vi "Begin.vi"(8 "error in":errorcluster) -> (0 "error out":errorcluster)   [LabVIEW 2014]
doc: "Called before other user functions, this VI is expected to open initial I/O refnums, load in file data, and do all program initialization. Notice that the <B>error out</B> terminal is simply used for data flow. Wiring it to other structures or subVIs ensures that this VI runs first."
uses:
  <vilib>/Rock Robotics/WPI/SafetyOutput/WPI_SafetyOutputConfigMenu.ctl
  <vilib>/Rock Robotics/WPI/DriverStation/WPI_DriverStationRobotMode2.ctl
  <vilib>/Rock Robotics/WPI/Joystick/WPI_JoystickDeviceEnum.ctl
  <vilib>/Rock Robotics/SystemInterfaces/DIO/FPGA_DIOPWMChannel.ctl
  <vilib>/Rock Robotics/WPI/Solenoid/WPI_SolenoidChannel.ctl
  navX-MXP Library/COMMON/TypeDefs/Value TypeDefs/navX Update Rate.ctl
  navX-MXP Library/COMMON/TypeDefs/Value TypeDefs/navX Interface Protocol.ctl
  <vilib>/Rock Robotics/SystemInterfaces/i2clib/i2c_bus.ctl
  <vilib>/Rock Robotics/SystemInterfaces/DIO/FPGA_DIOChannel.ctl
  <vilib>/Rock Robotics/WPI/Solenoid/WPI_SolenoidValue.ctl
  Robot Global Data.vi
  <vilib>/Rock Robotics/Network Tables/SD Write String Array.vi
  <vilib>/Rock Robotics/WPI/RobotDrive/WPI_RobotDriveOpen4MotorWithTalon.vi
  <vilib>/Rock Robotics/WPI/Solenoid/WPI_SolenoidOpenDouble.vi
  <vilib>/Rock Robotics/WPI/MotorControl/WPI_MotorControlOpen Talon.vi
  <vilib>/Rock Robotics/WPI/Solenoid/WPI_SolenoidSetEnum.vi
  navX-MXP Library/navX-MXP IMU.lvlib
panel:
  out "North":dbl
  out "Opened?":bool
  # "EDITED: 3/8/15"
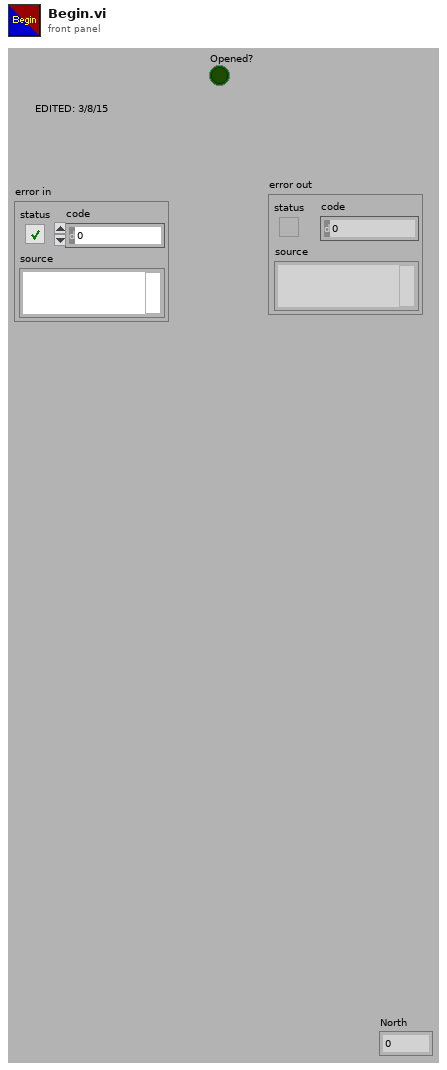
[diagram p1: front panel]
types:
  T1 = typedef "WPI_SolenoidValue.ctl" = enum16{"Off", "On", "Forward", "Reverse"}
  T2 = typedef "WPI_SolenoidChannel.ctl" = enum8{"Solenoid 0", "Solenoid 1", "Solenoid 2", "Solenoid 3", "Solenoid 4", "Solenoid 5", "Solenoid 6", "Solenoid 7", "Invalid"}
  T3 = typedef "FPGA_DIOPWMChannel.ctl" = enum8{"PWM 0", "PWM 1", "PWM 2", "PWM 3", "PWM 4", "PWM 5", "PWM 6", "PWM 7", "PWM 8", "PWM 9", "PWM MXP 0", "PWM MXP 1", "PWM MXP 2", "PWM MXP 3", "PWM MXP 4", "PWM MXP 5", "PWM MXP 6", "PWM MXP 7", "PWM MXP 8", "PWM MXP 9", "Invalid"}
  T4 = typedef "WPI_JoystickDeviceEnum.ctl" = enum16{"USB 0", "USB 1", "USB 2", "USB 3", "USB 4", "USB 5"}
  T5 = typedef "FPGA_DIOChannel.ctl" = enum8{"DIO 0", "DIO 1", "DIO 2", "DIO 3", "DIO 4", "DIO 5", "DIO 6", "DIO 7", "DIO 8", "DIO 9", "DIO MXP 0", "DIO MXP 1", "DIO MXP 2", "DIO MXP 3", "DIO MXP 4", "DIO MXP 5", "DIO MXP 6", "DIO MXP 7", "DIO MXP 8", "DIO MXP 9", "DIO MXP 10", "DIO MXP 11", "DIO MXP 12", "DIO MXP 13", "DIO MXP 14", "DIO MXP 15", "Invalid"}
  T6 = typedef "i2c_bus.ctl" = enum16{"I2C On-Board", "I2C MXP", "Invalid"}
  T7 = typedef "navX-MXP IMU.lvlib/navX Interface Protocol.ctl" = enum16{"SPI", "I2C"}
  T8 = typedef "navX-MXP IMU.lvlib/navX Update Rate.ctl" = u8
  T9 = typedef "WPI_DriverStationRobotMode2.ctl" = enum16{"Autonomous Disabled", "Autonomous Enabled", "Teleop Disabled", "Teleop Enabled", "Disconnected", "Finish", "Test Disabled", "Test Enabled", "Emergency Stopped"}
  T10 = typedef "WPI_SafetyOutputConfigMenu.ctl" = enum16{"Enable", "Disable"}
  T11 = typedef "WPI_JoystickDevRef.ctl" = cluster{"Device":T4}
  T12 = typedef "WPI_RobotDriveDevRef.ctl" = cluster{"DevStatus":errorcluster, "Motors[]":T13[], "Square Inputs":bool, "Max Output":dbl}
  T13 = typedef "WPI_MotorControlDeviceRef.ctl" = cluster{"DeviceStatus":errorcluster, "Type":T14, "PWM":cluster{"Controller":T15, "PWM Channel":T3, "DeadBand":T16}, "CAN":cluster{"Device Number":u8, "Control Mode":T17, "Semaphore":T18, "Max Vout":dbl, "TalonSRX Control Mode":T19}, "Invert":bool, "TransformRef":T20, "InvTransformRef":T20}
  T14 = typedef "WPI_MotorControlType.ctl" = enum16{"PWM", "CAN", "CANTalonSRX"}
  T15 = typedef "FPGA_TypedefDigitalModule.ctl" = enum16{"Controller 1"}
  T16 = typedef "WPI_PWMDeadband.ctl" = cluster{"Name":string, "maxPositivePwm":i32, "minPositivePwm":i32, "centerPwm":i32, "maxNegativePwm":i32, "minNegativePwm":i32, "angularRange":u16}
  T17 = typedef "WPI_CANJaguar_ControlMode.ctl" = enum8{"Percent VBus", "Current", "Speed", "Position", "Voltage"}
  T18 = typedef "Semaphore RefNum" = refnum<k1>
  T19 = typedef "WPI_CANTalonSRX_APIControlMode.ctl" = enum8{"Percent VBus", "Speed", "Position", "Slave", "Unchanged / Invalid"}
  T20 = typedef "WPI_PWMTransform_ConPane.ctl" = refnum<vi>
  T21 = typedef "WPI_SolenoidDevRef.ctl" = cluster{"DevStatus":errorcluster, "Pneumatics Control Module":u8, "Forward Solenoid Channel":T2, "Reverse Solenoid Channel":T2}
  T22 = typedef "navX-MXP IMU.lvlib/navX Device TypeDef.ctl" = cluster{"navX Interface Protocol":T7, "navX Interface Protocol TypeDefs":cluster{"SPIDevRef":T23, "I2CDevRef":T25}, "navX System Information":cluster{"Board Information":T26, "Status":T27, "Offsets":T31}, "navX Common Information":cluster{"Update Rate (4Hz-60Hz)":T8, "refnum name":string, "error":errorcluster}}
  T23 = typedef "WPI_SPIDevRef.ctl" = cluster{"DevStatus":errorcluster, "Handle":i32, "Controller":T15, "SPI Bus":T24}
  T24 = typedef "spi_bus.ctl" = enum16{"SPI On-Board, CS0", "SPI On-Board, CS1", "SPI On-Board, CS2", "SPI On-Board, CS3", "SPI MXP", "Invalid"}
  T25 = typedef "WPI_I2CDevRef.ctl" = cluster{"DevStatus":errorcluster, "Controller":T15, "Device Address":u8, "Handle":i32, "I2C Bus":T6}
  T26 = typedef "navX-MXP IMU.lvlib/navX Board Information.ctl" = cluster{"WhoAmI (50 | 0x32)":u8, "Board Revision":u8, "Firmware Major Version":u8, "Firmware Minor Version":u8}
  T27 = typedef "navX-MXP IMU.lvlib/navX Status Data.ctl" = cluster{"Update Rate Hz":u8, "Accelerometer Full-Scale Range":u8, "Gyro Full-Scale Range":u16, "NAVX_OP_STATUS":T28, "NAVX_CAL_STATUS":T29, "NAVX_SELFTEST_STATUS":u8, "NAVX_SENSOR_STATUS":T30}
  T28 = typedef "navX-MXP IMU.lvlib/navX NAVX_OP_STATUS.ctl" = u8
  T29 = typedef "navX-MXP IMU.lvlib/navX NAVX_CAL_STATUS.ctl" = u8
  T30 = typedef "navX-MXP IMU.lvlib/navX NAVX_SENSOR_STATUS.ctl" = cluster{"MOVING":bool, "YAW_STABLE":bool, "MAG_DISTURBANCE":bool, "ALTITUDE_VALID":bool, "SEALEVEL_PRESS_SET":bool, "FUSED_HEADING_VALID":bool}
  T31 = typedef "navX-MXP IMU.lvlib/navX Offsets Data.ctl" = cluster{"Yaw":dbl, "Quat W":dbl, "Quat X":dbl, "Quat Y":dbl, "Quat Z":dbl}
  T32 = typedef "WPI_DigitalInputDevRef.ctl" = cluster{"DevStatus":errorcluster, "DIO Channel":T5, "Controller":T15}
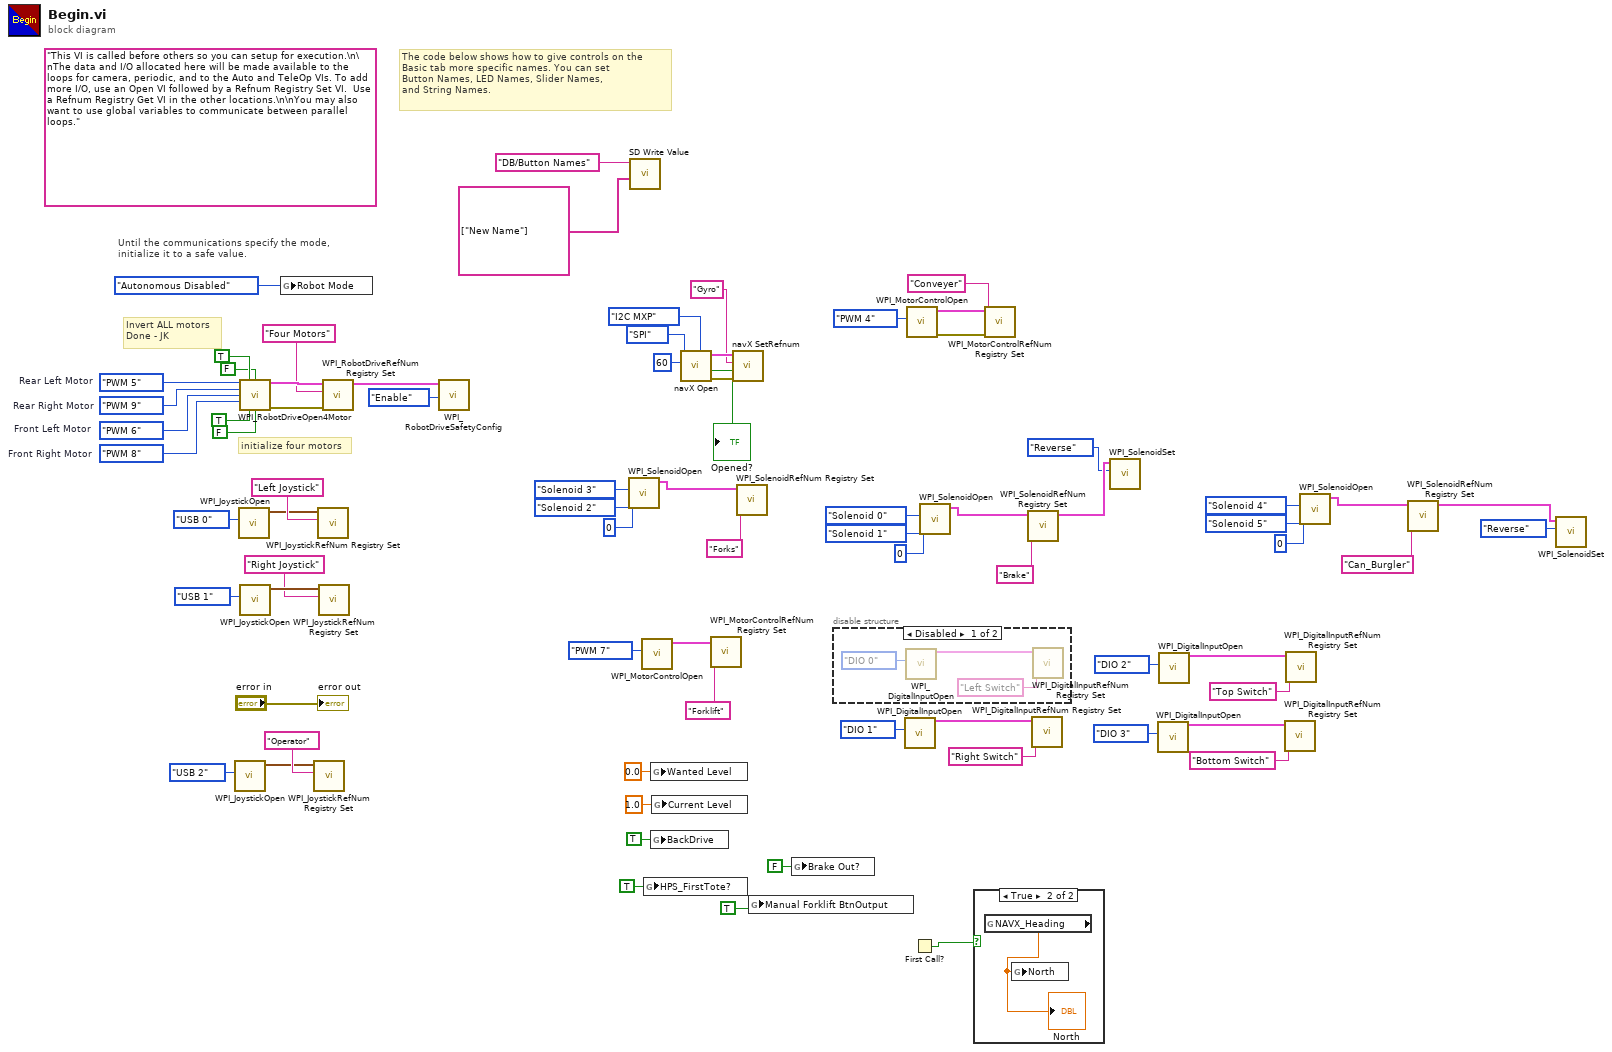
[diagram p0: block diagram]
diagram:
  w63 = FPGA_DIOPWMChannel."PWM 8"  # Front Right Motor
  w64 = FPGA_DIOPWMChannel."PWM 6"  # Front Left Motor
  w65 = FPGA_DIOPWMChannel."PWM 9"  # Rear Right Motor
  w66 = FPGA_DIOPWMChannel."PWM 5"  # Rear Left Motor
  (unwired) "This VI is called before others so you can setup for execution.\n\nThe data and I/O allocated here will be made available to the loops for camera, periodic, and to the Auto and TeleOp VIs. To add more I/O, use an Open VI followed by a Refnum Registry Set VI.  Use a Refnum Registry Get VI in the other locations.\n\nYou may also want to use global variables to communicate between parallel loops."
  # "Invert ALL motors\nDone - JK"
  # "The code below shows how to give controls on the\nBasic tab more specific names. You can set\nButton Names, LED Names, Slider Names,\nand String Names."
  # "Until the communications specify the mode,\ninitialize it to a safe value."
  # "initialize four motors"
  n1 = call <vilib>:"WPI_JoystickOpen.vi"("JoystickDevice"=WPI_JoystickDeviceEnum."USB 2") -> ("JoystickDevRef"=w15:T11)  [unwired: 10 in]
  n2 = call <vilib>:"WPI_JoystickOpen.vi"("JoystickDevice"=WPI_JoystickDeviceEnum."USB 0") -> ("JoystickDevRef"=w68:T11)  [unwired: 10 in]
  n3 = call-poly <vilib>:"WPI_RobotDriveOpen4Motor.vi"("Rear Left Motor"=w66, "Rear Left Motor Inverted"=TRUE, "Rear Right Motor Inverted"=FALSE, "Rear Right Motor"=w65, "Front Left Motor"=w64, "Front Right Motor"=w63, "Front Left Motor Inverted"=TRUE, "Front Right Motor Inverted"=FALSE) -> ("RobotDriveDevRef"=w75:T12, "error out"=w73:errorcluster)  [unwired: 6 in]
  n4 = call <vilib>:"WPI_JoystickOpen.vi"("JoystickDevice"=WPI_JoystickDeviceEnum."USB 1") -> ("JoystickDevRef"=w35:T11)  [unwired: 10 in]
  n5 = global write "Robot Global Data.vi" "Robot Mode"(WPI_DriverStationRobotMode2."Autonomous Disabled" ("Robot Mode")) -> ()
  n6 = call <vilib>:"WPI_JoystickRefNum Registry Set.vi"("refnum name"="Operator", "JoystickDevRef"=w15) -> ()  [unwired: 8 in, 2 out]
  n7 = call <vilib>:"WPI_JoystickRefNum Registry Set.vi"("refnum name"="Left Joystick", "JoystickDevRef"=w68) -> ()  [unwired: 8 in, 2 out]
  n8 = call <vilib>:"WPI_JoystickRefNum Registry Set.vi"("refnum name"="Right Joystick", "JoystickDevRef"=w35) -> ()  [unwired: 8 in, 2 out]
  n9 = call <vilib>:"WPI_RobotDriveRefNum Registry Set.vi"("error in (no error)"=w73, "refnum name"="Four Motors", "RobotDriveDevRef"=w75) -> ("RobotDriveDevRef"=w72:T12)  [unwired: 8 out]
  n10 = call <vilib>:"WPI_RobotDriveSafetyConfig.vi"("mode"=WPI_SafetyOutputConfigMenu."Enable", "RobotDriveDevRef"=w72) -> ()  [unwired: 8 in, 2 out]
  n11 = call-poly <vilib>:"WPI_SolenoidOpen.vi"("Reverse Solenoid Channel"=WPI_SolenoidChannel."Solenoid 2", "Forward Solenoid Channel"=WPI_SolenoidChannel."Solenoid 3", "Pneumatics Control Module (0)"=u8 0) -> ("SolenoidDevRef"=w55:T21)  [unwired: 7 in, 1 out]
  n12 = call-poly <vilib>:"SD Write Value.vi"("String Array"=string[] ["New Name"], "Name"="DB/Button Names") -> ()  [unwired: 8 in, 2 out]
  n13 = call-poly <vilib>:"WPI_MotorControlOpen.vi"("PWM Channel"=FPGA_DIOPWMChannel."PWM 7") -> ("MotorControlDeviceRef"=w38:T13)  [unwired: 9 in, 1 out]
  n14 = global write "Robot Global Data.vi" "HPS_FirstTote?"(TRUE ("HPS_FirstTote?")) -> ()
  n15 = global write "Robot Global Data.vi" "Wanted Level"(0.0 ("Wanted Level")) -> ()
  n16 = global write "Robot Global Data.vi" "BackDrive"(TRUE ("BackDrive")) -> ()
  n17 = global write "Robot Global Data.vi" "Current Level"(1.0 ("Current Level")) -> ()
  n18 = call "navX Open.vi"("I2C Bus"=i2c_bus."I2C MXP", "Update Rate (4Hz-60Hz)"=T8 60, "navX Interface Protocol"=navX_Interface_Protocol."SPI") -> ("error out"=w48:errorcluster, "Opened?"=→"Opened?":bool, "navX Device TypeDef"=w47:T22)  [unwired: 6 in]
  n19 = call <vilib>:"WPI_MotorControlRefNum Registry Set.vi"("refnum name"="Forklift", "MotorControlDevRef"=w38) -> ()  [unwired: 8 in, 2 out]
  n20 = call "navX SetRefnum.vi"("error in (no error)"=w48, "refnum name"="Gyro", "navX Device TypeDef"=w47) -> ()  [unwired: 7 in, 2 out]
  n21 = call <vilib>:"WPI_SolenoidRefNum Registry Set.vi"("refnum name"="Forks", "SolenoidDevRef"=w55) -> ()  [unwired: 8 in, 2 out]
  n22 = global write "Robot Global Data.vi" "Manual Forklift BtnOutput"(TRUE ("Brake Out?")) -> ()
  n23 = global write "Robot Global Data.vi" "Brake Out?"(FALSE ("Brake Out?")) -> ()
  n24 = disable-structure shown="Disabled" {
    frame Disabled {
      n25 = call <vilib>:"WPI_DigitalInputOpen.vi"("DIO Channel"=FPGA_DIOChannel."DIO 0") -> ("DigitalInputDevRef"=w77:T32)  [unwired: 9 in, 1 out]
      n26 = call <vilib>:"WPI_DigitalInputRefNum Registry Set.vi"("refnum name"="Left Switch", "DigitalInputDevRef"=w77) -> ()  [unwired: 8 in, 2 out]
    }
    frame Enabled {
    }
  }
  n27 = call <vilib>:"WPI_DigitalInputOpen.vi"("DIO Channel"=FPGA_DIOChannel."DIO 1") -> ("DigitalInputDevRef"=w32:T32)  [unwired: 9 in, 1 out]
  n28 = call-poly <vilib>:"WPI_MotorControlOpen.vi"("PWM Channel"=FPGA_DIOPWMChannel."PWM 4") -> ("error out"=w10:errorcluster, "MotorControlDeviceRef"=w11:T13)  [unwired: 9 in]
  n29 = First Call?() -> (First Call?: T/F=w8:bool)
  n30 = call-poly <vilib>:"WPI_SolenoidOpen.vi"("Reverse Solenoid Channel"=WPI_SolenoidChannel."Solenoid 1", "Forward Solenoid Channel"=WPI_SolenoidChannel."Solenoid 0", "Pneumatics Control Module (0)"=u8 0) -> ("SolenoidDevRef"=w40:T21)  [unwired: 7 in, 1 out]
  n31 = case shown="True" w8 {
    frame False {
    }
    frame True {
      n32 = global read "Robot Global Data.vi" "NAVX_Heading"() -> (w79:dbl)
      "North" <- w79
      n33 = global write "Robot Global Data.vi" "North"(w79) -> ()
    }
  }
  n34 = call <vilib>:"WPI_MotorControlRefNum Registry Set.vi"("error in (no error)"=w10, "refnum name"="Conveyer", "MotorControlDevRef"=w11) -> ()  [unwired: 7 in, 2 out]
  n35 = call <vilib>:"WPI_SolenoidRefNum Registry Set.vi"("refnum name"="Brake", "SolenoidDevRef"=w40) -> ("SolenoidDevRef"=w21:T21)  [unwired: 8 in, 1 out]
  n36 = call <vilib>:"WPI_DigitalInputRefNum Registry Set.vi"("refnum name"="Right Switch", "DigitalInputDevRef"=w32) -> ()  [unwired: 8 in, 2 out]
  n37 = call-poly <vilib>:"WPI_SolenoidSet.vi"("Value"=WPI_SolenoidValue."Reverse", "SolenoidDevRef"=w21) -> ()  [unwired: 8 in, 2 out]
  n38 = call <vilib>:"WPI_DigitalInputOpen.vi"("DIO Channel"=FPGA_DIOChannel."DIO 3") -> ("DigitalInputDevRef"=w29:T32)  [unwired: 9 in, 1 out]
  n39 = call <vilib>:"WPI_DigitalInputOpen.vi"("DIO Channel"=FPGA_DIOChannel."DIO 2") -> ("DigitalInputDevRef"=w26:T32)  [unwired: 9 in, 1 out]
  n40 = call <vilib>:"WPI_DigitalInputRefNum Registry Set.vi"("refnum name"="Bottom Switch", "DigitalInputDevRef"=w29) -> ()  [unwired: 8 in, 2 out]
  n41 = call <vilib>:"WPI_DigitalInputRefNum Registry Set.vi"("refnum name"="Top Switch", "DigitalInputDevRef"=w26) -> ()  [unwired: 8 in, 2 out]
  n42 = call-poly <vilib>:"WPI_SolenoidOpen.vi"("Reverse Solenoid Channel"=WPI_SolenoidChannel."Solenoid 5", "Forward Solenoid Channel"=WPI_SolenoidChannel."Solenoid 4", "Pneumatics Control Module (0)"=u8 0) -> ("SolenoidDevRef"=w3:T21)  [unwired: 7 in, 1 out]
  n43 = call <vilib>:"WPI_SolenoidRefNum Registry Set.vi"("refnum name"="Can_Burgler", "SolenoidDevRef"=w3) -> ("SolenoidDevRef"=w1:T21)  [unwired: 8 in, 1 out]
  n44 = call-poly <vilib>:"WPI_SolenoidSet.vi"("Value"=WPI_SolenoidValue."Reverse", "SolenoidDevRef"=w1) -> ()  [unwired: 8 in, 2 out]
  "error out" <- "error in"
